vi "Package Data.vi"(8 "error in":errorcluster, 10 "DataIn":string, 11 "M data in":refnum<class "M data.lvclass">) -> (0 "error out":errorcluster, 3 "M data out":refnum<class "M data.lvclass">)   [LabVIEW 2019, in "M data.lvclass"]
uses:
  M data.lvclass
  Z:/sw_repo/handix/source/Reusable/Data/Data.lvclass
  Z:/sw_repo/handix/source/Devices/Alicat/Session Based/Data/Alicat Data.lvclass
  M data.lvclass/M data.ctl
  Reusable/Data/Write measTime.vi
  Reusable/General/Atmospheric/Atmospheric Constants.vi
  Reusable/General/Atmospheric/Atmospheric Library.lvlib
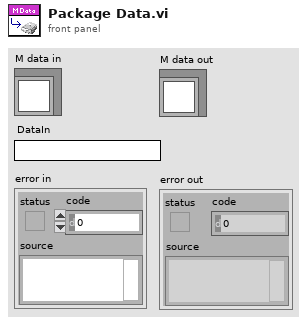
[diagram p1: front panel]
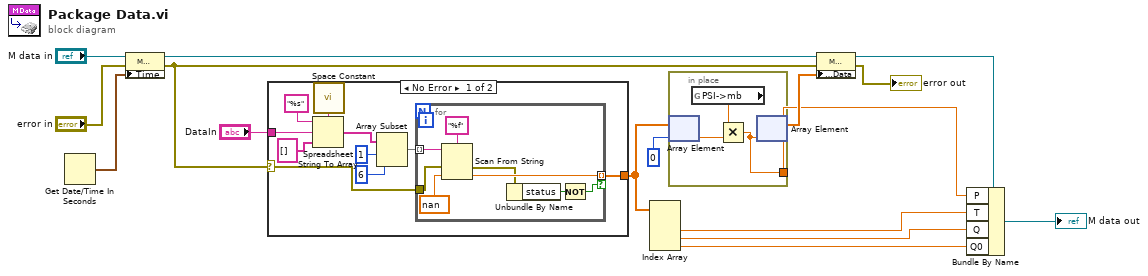
[diagram p0: block diagram]
diagram:
  n1 = Get Date/Time In Seconds() -> (seconds since 1Jan1904=w13:timestamp)
  n2 = property class="M Data"(reference="M data in", error in="error in", "Time"=w13) -> (reference out=w8:refnum<class "M data.lvclass">, error out=w2:errorcluster)
  n3 = case shown="No Error" w2 {
    selector: w2 -> [w17 _]
    tunnel: "DataIn" -> [w23 _]
    tunnel: [w19 _] -> w6
    frame No Error {
      n4 = call <vilib>:"Space Constant.vi"() -> ("String"=w25:string)
      n5 = Spreadsheet String To Array(delimiter (Tab)=w25, format string="%s", spreadsheet string=w23, array type (2D Dbl)=string[] []) -> (array=w22:string[])
      n6 = Array Subset(array=w22, index=1, length=6) -> (w20:string[])
      n7 = for {
        tunnel: w20 -> [w31] mode=indexing
        tunnel: [w32] -> w19 mode=indexing if=w28
        tunnel: w17 -> [w27]
        n8 = Scan From String(format string="%f", input string=w31, error in=w27, default 1=sgl nan ("default value 1")) -> (error out=w30:errorcluster, output 1=w32:sgl)  [unwired: 1 in, 2 out]
        n9 = Unbundle By Name(w30) -> ("status"=w29:bool)
        n10 = Not(x=w29) -> (.not. x?=w28:bool)
      }
    }
    frame Error {
    }
  }
  n11 = Index Array(array=w6) -> (element #2=w16:sgl, element #3=w15:sgl, element #4=w14:sgl)  [unwired: 4 in, 1 out]
  n12 = in-place {
    in-place-border: [w35] -> w3
    n13 = in-place-array #1(w6, 0) -> (w36:sgl)
    n14 = global read "Atmospheric Constants.vi" "PSI->mb"() -> (w37:sgl)
    n15 = Multiply(x=w37, y=w36) -> (x*y=w35:sgl)
    n16 = in-place-array #1(w35) -> (w4:sgl[])  [unwired: 1 out]
  }
  n17 = property class="M Data"(reference=w8, error in=w2, "Accessors:Data"=w4) -> (reference out=w7:refnum<class "M data.lvclass">, error out=→"error out":errorcluster)
  n18 = Bundle By Name(cluster=w7, "P"=w3, "T"=w16, "Q"=w15, "Q0"=w14) -> (→"M data out":refnum<class "M data.lvclass">)
